vi "JKI SM Editor - Fix Bad VI.vi"(8 "error in (no error)":errorcluster, 11 "Output Package File Path":path) -> (0 "error out":errorcluster)   [LabVIEW 2020]
uses:
  <userlib>/_OpenG.lib/lvzip/lvzip.llb/ZLIB Open ZIP Mode__ogtk.ctl
  <userlib>/_OpenG.lib/lvzip/lvzip.llb/subVI/ZLIB Extract All Files To Dir (Path)__ogtk.vi
  <userlib>/_OpenG.lib/file/file.llb/Convert File Extension (Path)__ogtk.vi
  <userlib>/_OpenG.lib/lvzip/lvzip.llb/subVI/ZLIB Compress Directory (Path)__ogtk.vi
  <userlib>/_OpenG.lib/file/file.llb/openg_file.lvlib
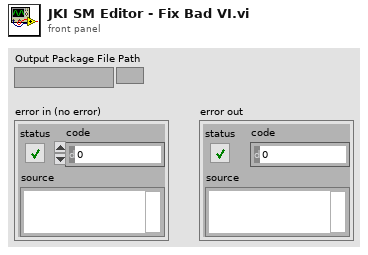
[diagram p1: front panel]
types:
  T1 = typedef "ZLIB Open ZIP Mode__ogtk.ctl" = enum16{"create new", "append to end", "append to archive"}
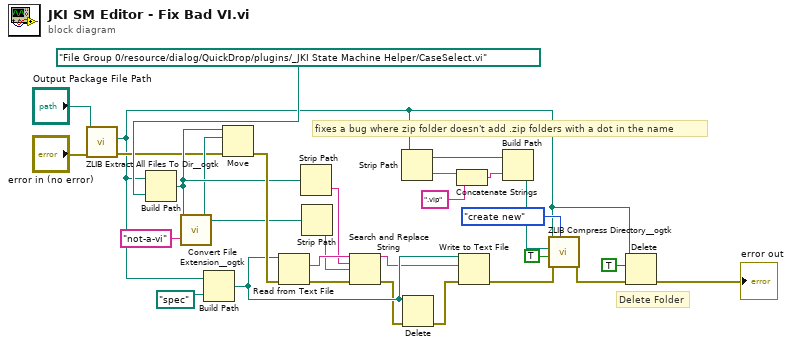
[diagram p0: block diagram]
diagram:
  # "Delete Folder"
  # "fixes a bug where zip folder doesn't add .zip folders with a dot in the name"
  n1 = call-poly <userlib>:"ZLIB Extract All Files To Dir__ogtk.vi"("error in (no error)"="error in (no error)", "archive name (file dialog)"="Output Package File Path") -> ("error out"=w15:errorcluster, "destination directory out"=w3:path)  [unwired: 7 in, 1 out]
  n2 = Build Path(base path=w3, name or relative path=path "File Group 0/resource/dialog/QuickDrop/plugins/_JKI State Machine Helper/CaseSelect.vi" ("base path")) -> (appended path=w19:path)
  n3 = call-poly <userlib>:"Convert File Extension__ogtk.vi"("new ending (none)"="not-a-vi", "file name"=w19) -> ("new filename"=w18:path)  [unwired: 1 out]
  n4 = Build Path(base path=w3, name or relative path=path "spec" ("base path")) -> (appended path=w26:path)
  n5 = Move(source path=w19, error in=w15, 10:w18) -> (error out=w27:errorcluster)  [unwired: 2 in, 2 out]
  n6 = Read from Text File(file (use dialog)=w26, error in=w27) -> (text=w22:string, error out=w17:errorcluster)  [unwired: 2 in, 2 out]
  n7 = Strip Path(path=w19) -> (name=w20:string)  [unwired: 1 out]
  n8 = Strip Path(path=w18) -> (name=w21:string)  [unwired: 1 out]
  n9 = Search and Replace String(input string=w22, search string=w20, replace string=w21, error in=w17) -> (result string=w23:string, error out=w24:errorcluster)  [unwired: 4 in, 2 out]
  n10 = Strip Path(path=w3) -> (stripped path=w9:path, name=w8:string)
  n11 = Delete(path (use dialog)=w26, error in=w24) -> (error out=w25:errorcluster)  [unwired: 3 in, 2 out]
  n12 = Concatenate Strings(w8, ".vip" ("string")) -> (w7:string)
  n13 = Write to Text File(file (use dialog)=w26, text=w23, error in=w25) -> (error out=w12:errorcluster)  [unwired: 1 in, 2 out]
  n14 = Build Path(base path=w9, name or relative path=w7) -> (appended path=w5:path)
  n15 = call-poly <userlib>:"ZLIB Compress Directory__ogtk.vi"("append (create new)"=ZLIB_Open_ZIP_Mode__ogtk."create new", "error in (no error)"=w12, "include subdirectories (F)"=TRUE, "archive name (root directory with .zip ending)"=w5, "root directory (file dialog)"=w3) -> ("error out"=w2:errorcluster)  [unwired: 4 in, 2 out]
  n16 = Delete(path (use dialog)=w3, entire hierarchy (F)=TRUE, error in=w2) -> (error out=→"error out":errorcluster)  [unwired: 2 in, 2 out]
